vi "Send Message Array.vi"(8 "error in (no error)":errorcluster, 10 "Message Array":T1[](array[typedef]), 11 "Producer in":refnum<class "Abstract Producer.lvclass">) -> (0 "error out":errorcluster, 3 "Producer out":refnum<class "Abstract Producer.lvclass">)   [LabVIEW 2017, in "Routing and Faulting Engine.lvlib"]
uses:
  Routing and Faulting Engine.lvlib
  Producer Message.ctl
  Includes/CDMessaging.lvlibp/Message/Abstract Message/Abstract Message.lvclass
  Includes/CDMessaging.lvlibp/Producer/Abstract Producer/Abstract Producer.lvclass
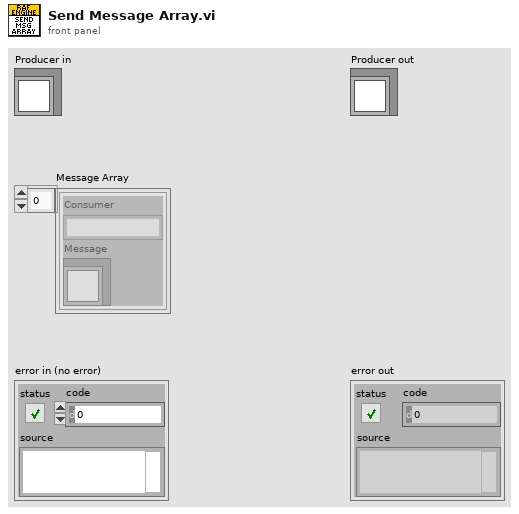
[diagram p1: front panel]
types:
  T1 = typedef "Routing and Faulting Engine.lvlib/Producer Message.ctl" = cluster{"Consumer":string, "Message":refnum<class "Abstract Message.lvclass">}
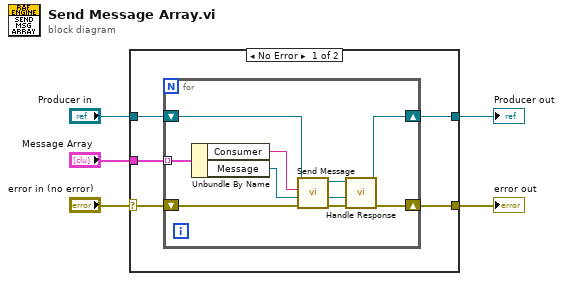
[diagram p0: block diagram]
diagram:
  n1 = case shown="No Error" "error in (no error)" {
    selector: "error in (no error)" -> [w6 w22]
    tunnel: [w10 w22] -> w5
    tunnel: "Producer in" -> [w9 w21]
    tunnel: "Message Array" -> [w8 _]
    tunnel: [w7 w21] -> w2
    frame No Error {
      n2 = for {
        shift-right: [w11] -> w10
        shift-left: w6 -> [w20]
        shift-right: [w12] -> w7
        shift-left: w9 -> [w19]
        tunnel: w8 -> [w18] mode=indexing
        n3 = Unbundle By Name(w18) -> ("Consumer"=w17:string, "Message"=w16:refnum<class "Abstract Message.lvclass">)
        n4 = call-dynamic "Send Message.vi"("error in (no error)"=w20, "Message in"=w16, "Consumer in"=w17, "Abstract Producer in"=w19) -> ("error out"=w15:errorcluster, "Message out"=w14:refnum<class "Abstract Message.lvclass">, "Abstract Producer out"=w13:refnum<class "Abstract Producer.lvclass">)  [unwired: 5 in]
        n5 = call-dynamic "Handle Response.vi"("error in (no error)"=w15, "Abstract Response Message"=w14, "Abstract Producer in"=w13) -> ("error out"=w11:errorcluster, "Abstract Producer out"=w12:refnum<class "Abstract Producer.lvclass">)  [unwired: 7 in]
      }
    }
    frame Error {
    }
  }
  "error out" <- w5
  "Producer out" <- w2
